vi "ack_bit.vi"(8 "Min Time SCL High":u32 caption="Count(uSec)", 9 "Min time SCL Low":u32 caption="Count(uSec)", 11 "ack":bool) -> ()   [LabVIEW 2019]
uses:
  <vilib>/rvi/eio/common/nirviEmuTemplateMethod_errors.vi
  <vilib>/eio/EIOMethodNode/EIOMethodNode.xnode
  <vilib>/eio/EIONode/EIONode.xnode
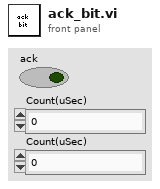
[diagram p1: front panel]
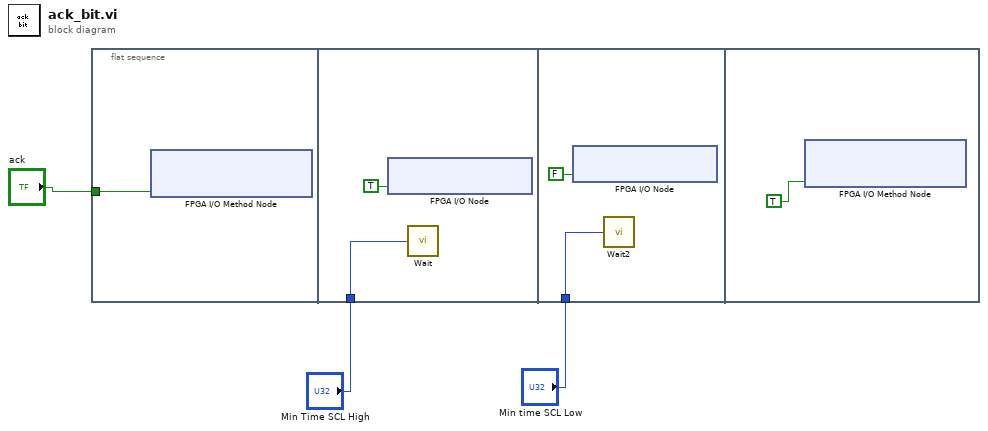
[diagram p0: block diagram]
diagram:
  n1 = flat-sequence {
    tunnel: "ack" -> [w4]
    tunnel: "Min Time SCL High" -> [w5]
    tunnel: "Min time SCL Low" -> [w7]
    frame #0 {
      n2 = xnode "FPGA I/O Method Node"("Enable"=w4) -> ()  [unwired: 1 in, 1 out]
    }
    frame #1 {
      n3 = xnode "FPGA I/O Node"("ConnectorA/DIO14"=TRUE) -> ()  [unwired: 1 in, 1 out]
      n4 = call "Wait"("Count(uSec)"=w5) -> ()  [unwired: 1 out]
    }
    frame #2 {
      n5 = xnode "FPGA I/O Node"("ConnectorA/DIO14"=FALSE) -> ()  [unwired: 1 in, 1 out]
      n6 = call "Wait2"("Count(uSec)"=w7) -> ()  [unwired: 1 out]
    }
    frame #3 {
      n7 = xnode "FPGA I/O Method Node"("Enable"=TRUE) -> ()  [unwired: 1 in, 1 out]
    }
  }
